vi "CreateEventsForStatus.vi"() -> (2 "Event Registration Refnum":refnum<event-registration>, 3 "Events":T1)   [LabVIEW 2019, in "SolutionBuilder.lvlib"]
uses:
  SolutionBuilder/SolutionBuilder.lvlib
  EventUpdateList.ctl
  EventItemBuilt.ctl
  SolutionBuilder/Events.ctl
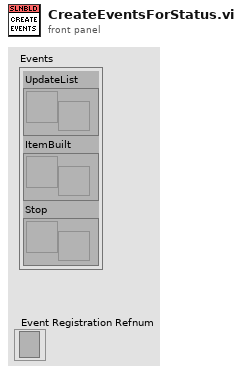
[diagram p1: front panel]
types:
  T1 = typedef "SolutionBuilder.lvlib/Events.ctl" = cluster{"UpdateList":T2, "ItemBuilt":T3, "Stop":refnum<user-event>}
  T2 = typedef "SolutionBuilder.lvlib/EventUpdateList.ctl" = refnum<user-event>
  T3 = typedef "SolutionBuilder.lvlib/EventItemBuilt.ctl" = refnum<user-event>
  T4 = cluster{"Item":string, "Project":string, "Result":string}
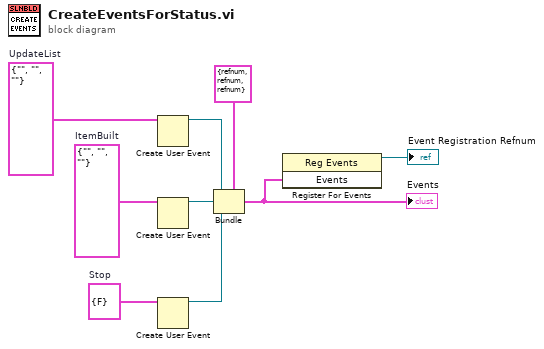
[diagram p0: block diagram]
diagram:
  w9 = T4 {"Item"="", "Project"="", "Result"=""}  # UpdateList
  w8 = cluster{"Stop":bool} {"Stop"=FALSE}  # Stop
  w7 = T4 {"Item"="", "Project"="", "Result"=""}  # ItemBuilt
  n1 = Create User Event(user event datatype=w9) -> (user event=w2:refnum<user-event>)  [unwired: 1 in, 1 out]
  n2 = Create User Event(user event datatype=w7) -> (user event=w1:refnum<user-event>)  [unwired: 1 in, 1 out]
  n3 = Create User Event(user event datatype=w8) -> (user event=w6:refnum<user-event>)  [unwired: 1 in, 1 out]
  n4 = Bundle(cluster=T1 {"UpdateList"=refnum, "ItemBuilt"=refnum, "Stop"=refnum} ("Events"), "UpdateList"=w2, "ItemBuilt"=w1, "Stop"=w6) -> (w4:T1)
  "Events" <- w4
  n5 = register-events(w4) -> (reference out=→"Event Registration Refnum":refnum<event-registration>)  [unwired: 2 in, 1 out]
